vi "Get filepath.vi"(8 "error in (no error)":errorcluster, 11 "DAQOrcaFlash in":refnum<class "DAQOrcaFlash.lvclass">) -> (0 "error out":errorcluster, 2 "filepath out":path, 3 "DAQOrcaFlash out":refnum<class "DAQOrcaFlash.lvclass">)   [LabVIEW 2012, in "DAQOrcaFlash.lvclass"]
uses:
  DAQOrcaFlash.lvclass
  DAQOrcaFlash.lvclass/DAQOrcaFlash.ctl
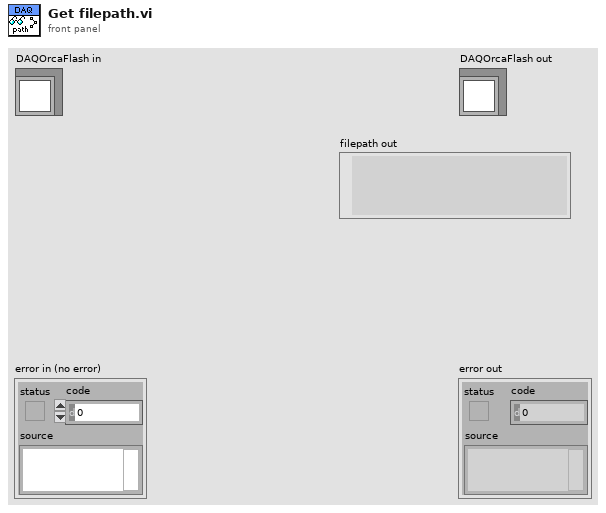
[diagram p1: front panel]
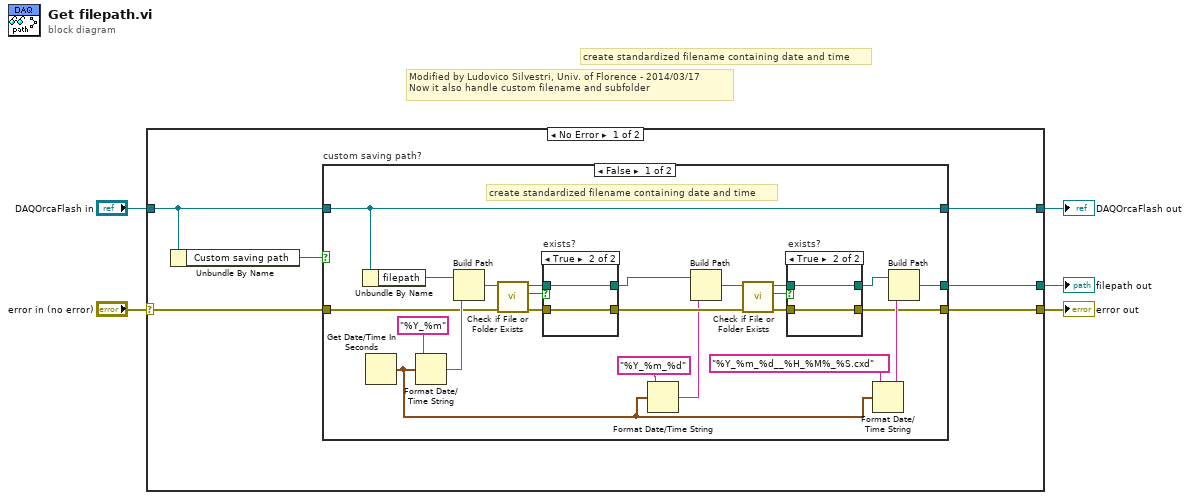
[diagram p0: block diagram]
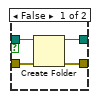
[diagram p2: hidden frame]
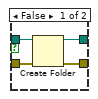
[diagram p3: hidden frame]
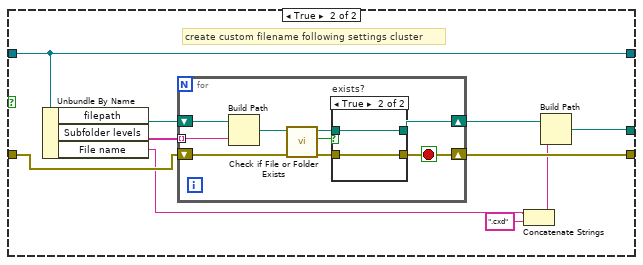
[diagram p4: hidden frame]
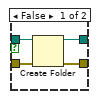
[diagram p5: hidden frame]
diagram:
  # "create standardized filename containing date and time"
  # "Modified by Ludovico Silvestri, Univ. of Florence - 2014/03/17\nNow it also handle custom filename and subfolder"
  n1 = case shown="No Error" "error in (no error)" {
    selector: "error in (no error)" -> [w11 w73]
    tunnel: [w10 w73] -> w4
    tunnel: [w6 w72] -> w3
    tunnel: "DAQOrcaFlash in" -> [w8 w72]
    tunnel: [w9 _] -> w2
    frame No Error {
      n2 = Unbundle By Name(w8) -> ("Custom saving path"=w7:bool)
      n3 = case "custom saving path?" shown="False" w7 {
        tunnel: w11 -> [w18 w50]
        tunnel: w8 -> [w13 w56]
        tunnel: [w15 w51] -> w10
        tunnel: [w12 w52] -> w9
        tunnel: [w13 w56] -> w6
        frame False {
          # "create standardized filename containing date and time"
          n4 = Unbundle By Name(w13) -> ("filepath"=w25:path)
          n5 = Get Date/Time In Seconds() -> (seconds since 1Jan1904=w17:timestamp)
          n6 = Format Date/Time String(time format string (%c)="%Y_%m", seconds (now)=w17) -> (date/time string=w19:string)  [unwired: 1 in]
          n7 = Build Path(base path=w25, name or relative path=w19) -> (appended path=w21:path)
          n8 = call <vilib>:"Check if File or Folder Exists.vi"("error in (no error)"=w18, "path"=w21) -> ("error out"=w24:errorcluster, "file or folder exists?"=w22:bool, "dup path"=w23:path)  [unwired: 7 in]
          n9 = case "exists?" shown="True" w22 {
            tunnel: w23 -> [w43 w45]
            tunnel: w24 -> [w44 w46]
            tunnel: [w42 w45] -> w33
            tunnel: [w41 w46] -> w32
            frame False {
              n10 = Create Folder(path (use dialog)=w43, error in=w44) -> (created path=w42:path, error out=w41:errorcluster)  [unwired: 1 in, 1 out]
            }
            frame True {
            }
          }
          n11 = Format Date/Time String(time format string (%c)="%Y_%m_%d", seconds (now)=w17) -> (date/time string=w30:string)  [unwired: 1 in]
          n12 = Build Path(base path=w33, name or relative path=w30) -> (appended path=w26:path)
          n13 = call <vilib>:"Check if File or Folder Exists.vi"("error in (no error)"=w32, "path"=w26) -> ("error out"=w29:errorcluster, "file or folder exists?"=w27:bool, "dup path"=w28:path)  [unwired: 7 in]
          n14 = case "exists?" shown="True" w27 {
            tunnel: w28 -> [w37 w39]
            tunnel: w29 -> [w38 w40]
            tunnel: [w36 w39] -> w14
            tunnel: [w35 w40] -> w15
            frame False {
              n15 = Create Folder(path (use dialog)=w37, error in=w38) -> (created path=w36:path, error out=w35:errorcluster)  [unwired: 1 in, 1 out]
            }
            frame True {
            }
          }
          n16 = Format Date/Time String(time format string (%c)="%Y_%m_%d__%H_%M%_%S.cxd", seconds (now)=w17) -> (date/time string=w16:string)  [unwired: 1 in]
          n17 = Build Path(base path=w14, name or relative path=w16) -> (appended path=w12:path)
        }
        frame True {
          # "create custom filename following settings cluster"
          n18 = Unbundle By Name(w56) -> ("filepath"=w55:path, "Subfolder levels"=w54:string[], "File name"=w49:string)
          n19 = for {
            tunnel: w54 -> [w64] mode=indexing
            shift-right: [w58] -> w53
            shift-left: w55 -> [w65]
            shift-right: [w57] -> w51
            shift-left: w50 -> [w59]
            stop <- w57 stop-if-true
            n20 = Build Path(base path=w65, name or relative path=w64) -> (appended path=w60:path)
            n21 = call <vilib>:"Check if File or Folder Exists.vi"("error in (no error)"=w59, "path"=w60) -> ("error out"=w63:errorcluster, "file or folder exists?"=w61:bool, "dup path"=w62:path)  [unwired: 7 in]
            n22 = case "exists?" shown="True" w61 {
              tunnel: w62 -> [w68 w70]
              tunnel: w63 -> [w69 w71]
              tunnel: [w67 w70] -> w58
              tunnel: [w66 w71] -> w57
              frame False {
                n23 = Create Folder(path (use dialog)=w68, error in=w69) -> (created path=w67:path, error out=w66:errorcluster)  [unwired: 1 in, 1 out]
              }
              frame True {
              }
            }
          }
          n24 = Concatenate Strings(w49, ".cxd" ("string")) -> (w47:string)
          n25 = Build Path(base path=w53, name or relative path=w47) -> (appended path=w52:path)
        }
      }
    }
    frame Error {
    }
  }
  "error out" <- w4
  "DAQOrcaFlash out" <- w3
  "filepath out" <- w2
